vi "Delete Items.vi"(8 "error in (no error)":errorcluster, 10 "Tag":string, 11 "reference":refnum<vi>) -> (0 "error out":errorcluster, 3 "reference out":refnum<vi>)   [LabVIEW 2019, in "Tree Control.lvlib"]
doc: "Delete Items in a Tree Control."
uses:
  Tree Control.lvlib
panel:
  # "No tag = delete all"
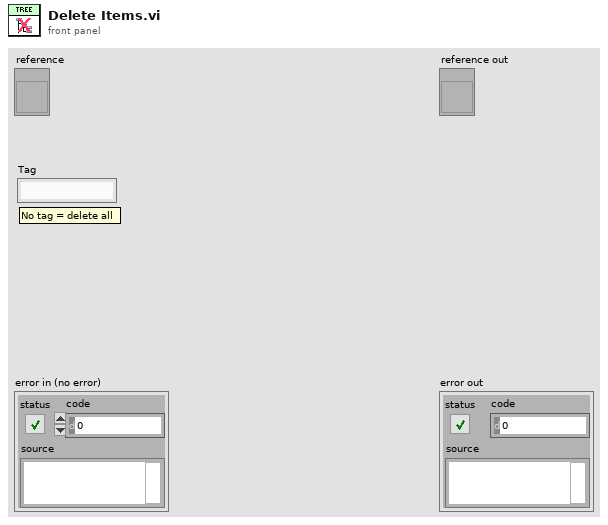
[diagram p1: front panel]
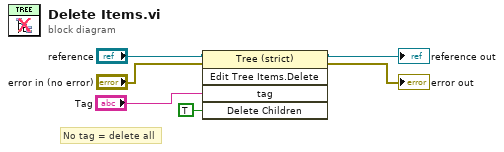
[diagram p0: block diagram]
diagram:
  # "No tag = delete all"
  n1 = invoke on="Invoke Node" class="Tree (strict)" method="Edit Tree Items.Delete"(reference="reference", error in="error in (no error)", "tag"="Tag", "Delete Children"=TRUE ("Delete Children?")) -> (reference out=→"reference out":refnum<vi>, error out=→"error out":errorcluster)  [unwired: 1 in, 3 out]
